vi "PicoScope3000aExampleBlockMSO_MultipleDevices.vi"() -> ()   [LabVIEW 2010]
uses:
  shared/PicoBuffers.ctl
  shared/Buffer and Transfer Settings.ctl
  shared/Acquisition Settings.ctl
  PicoScope3000aLib/PicoScope3000aDigitalChannelSettings.ctl
  PicoScope3000aLib/PicoScope3000aAnalogChannelSettings.ctl
panel:
  out "Overflow":i16[](array[numeric])
  in  "Serial Numbers":string[](array[string])
  out "Device Info":T1(array[cluster])
  out "Properties panel":T2(array[cluster]) {"Sample Frequency" format="%#_4p"; "Sample Rate" format="%#_4p"; "Max Samples Available" format="%#_4p"; "Number of Samples" format="%#_4p"; "Total Capture Time (sec)" format="%#_4p"; "Max Total Capture Time Available (sec)" format="%#_4p"}
  in  "Use Serial Numbers":bool
  in  "Scope Index":i32
  in  "Trigger Settings":T3={"Trigger Enabled"=FALSE, "Trigger Source"=enum."Channel A", "Trigger Threshold (volts)"=0.0, "Trigger Direction"=2, "Trigger Delay (samples)"=0, "Auto Trigger Time (ms)"=1000} {"Trigger Direction" items=["Above", "Below", "Rising", "Falling", "Rising or Falling"]}
  in  "Channel A Settings":T4={"Enabled"=TRUE, "Coupling"=1, "Range"=6, "Analogue Offset"=0.0, "Bandwidth Limit"=0} {"Bandwidth Limit" items=["Full", "20MHz"]; "Range" items=["10 mV", "20 mV", "50 mV", "100 mV", "200 mV", "500 mV", "1 V", "2 V", "5 V", "10 V", "20 V", "50 V ", "100 V"]; "Coupling" items=["AC", "DC"]}
  in  "Port 0 Settings":T5={"Enabled"=FALSE, "Logic Level"=9830} {"Logic Level" items=["1.5V TTL"=9830, "2.5V CMOS"=16383]}
  in  "Apply Settings":bool
  out "USB 3.0 device on non-USB 3.0 Port":bool=TRUE
  out "USB Powered":bool=TRUE
  out "error out":errorcluster
  in  "Buffer and Transfer Settings":T6={"startIndex"=0, "Samples"=100000, "Down Sample Ratio"=1, "Down-Sample Mode"=0} {"Down-Sample Mode" items=["RAW none"=2147483648, "None"=0, "Aggregate"=1, "Decimate"=2, "Average"=4]; "Down Sample Ratio" step=1; "Samples" format="%_6p"}
  in  "Acquisition Settings":T7={"preTriggerSamples"=0, "postTriggerSamples"=100000, "timebase"=10} {"postTriggerSamples" format="%_6p"; "preTriggerSamples" format="%_6p"}
  in  "stop":bool
  out "Scope \"N\"":cluster{i32, sgl, "Data":dbl[]}[](graph)
  in  "error in (no error)":errorcluster
  # "Bit 0 = ChA"
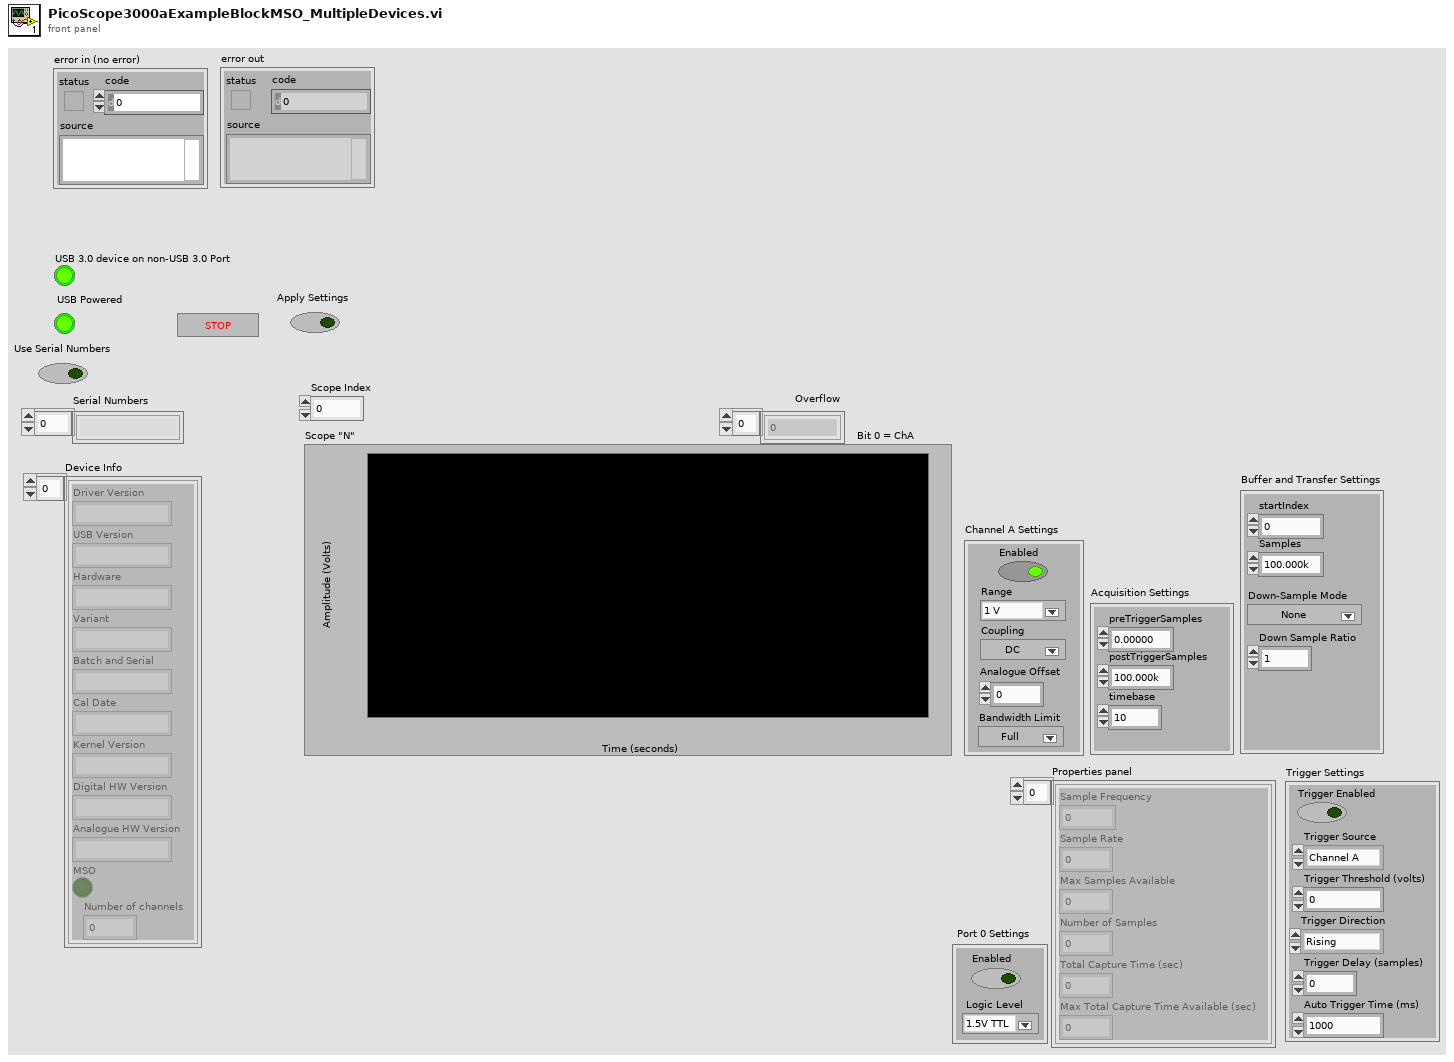
[diagram p1: front panel]
types:
  T1 = cluster{"Driver Version":string, "USB Version":string, "Hardware":string, "Variant":string, "Batch and Serial":string, "Cal Date":string, "Kernel Version":string, "Digital HW Version":string, "Analogue HW Version":string, "MSO":bool, "Number of channels":i16}[]
  T2 = cluster{"Sample Frequency":sgl, "Sample Rate":sgl, "Max Samples Available":i32, "Number of Samples":u32, "Total Capture Time (sec) ":sgl, "Max Total Capture Time Available (sec)":sgl}[]
  T3 = cluster{"Trigger Enabled":bool, "Trigger Source":enum32{"Channel A", "Channel B", "Channel C", "Channel D", "Ext."}, "Trigger Threshold (volts)":dbl, "Trigger Direction":u32, "Trigger Delay (samples)":u32, "Auto Trigger Time (ms)":i16}
  T4 = typedef "PicoScope3000aAnalogChannelSettings.ctl" = cluster{"Enabled":bool, "Coupling":u32, "Range":u32, "Analogue Offset":sgl, "Bandwidth Limit":u32}
  T5 = typedef "PicoScope3000aDigitalChannelSettings.ctl" = cluster{"Enabled":bool, "Logic Level":i16}
  T6 = typedef "Buffer and Transfer Settings.ctl" = cluster{"startIndex":u64, "Samples":u64, "Down Sample Ratio":u64, "Down-Sample Mode":u32}
  T7 = typedef "Acquisition Settings.ctl" = cluster{"preTriggerSamples":u64, "postTriggerSamples":u64, "timebase":u32}
  T8 = typedef "PicoBuffers.ctl" = cluster{"Max Buffer Pointers":u64[][][], "Min Buffer Pointers":u64[][][], "StreamingDataInfo":cluster{"Channel":u32, "Down-Sample Mode":u32, "PICO_DATA_TYPE":enum32{"PICO_INT8_T", "PICO_INT16_T", "PICO_INT32_T", "PICO_UINT32_T", "PICO_INT64_T", ""}, "Samples":i32, "bufferIndex":u64, "startIndex":i32, "overflow":i16}[][]}
  T9 = cluster{"Driver Version":string, "USB Version":string, "Hardware":string, "Variant":string, "Batch and Serial":string, "Cal Date":string, "Kernel Version":string, "Digital HW Version":string, "Analogue HW Version":string, "MSO":bool, "Number of channels":i16}
  T10 = cluster{"Sample Frequency":sgl, "Sample Rate":sgl, "Max Samples Available":i32, "Number of Samples":u32, "Total Capture Time (sec) ":sgl, "Max Total Capture Time Available (sec)":sgl}
  T11 = cluster{"Channel A Buffer":i16[], "Channel B Buffer":i16[], "Channel C Buffer":i16[], "Channel D Buffer":i16[], "Channel E Buffer":i16[], "Channel F Buffer":i16[], "Channel G Buffer":i16[], "Channel H Buffer":i16[], "Port 0 Buffer":i16[], "Port 1 Buffer":i16[]}[]
  T12 = cluster{"Channel A Buffer":i16[], "Channel B Buffer":i16[], "Channel C Buffer":i16[], "Channel D Buffer":i16[], "Channel E Buffer":i16[], "Channel F Buffer":i16[], "Channel G Buffer":i16[], "Channel H Buffer":i16[], "Port 0 Buffer":i16[], "Port 1 Buffer":i16[]}
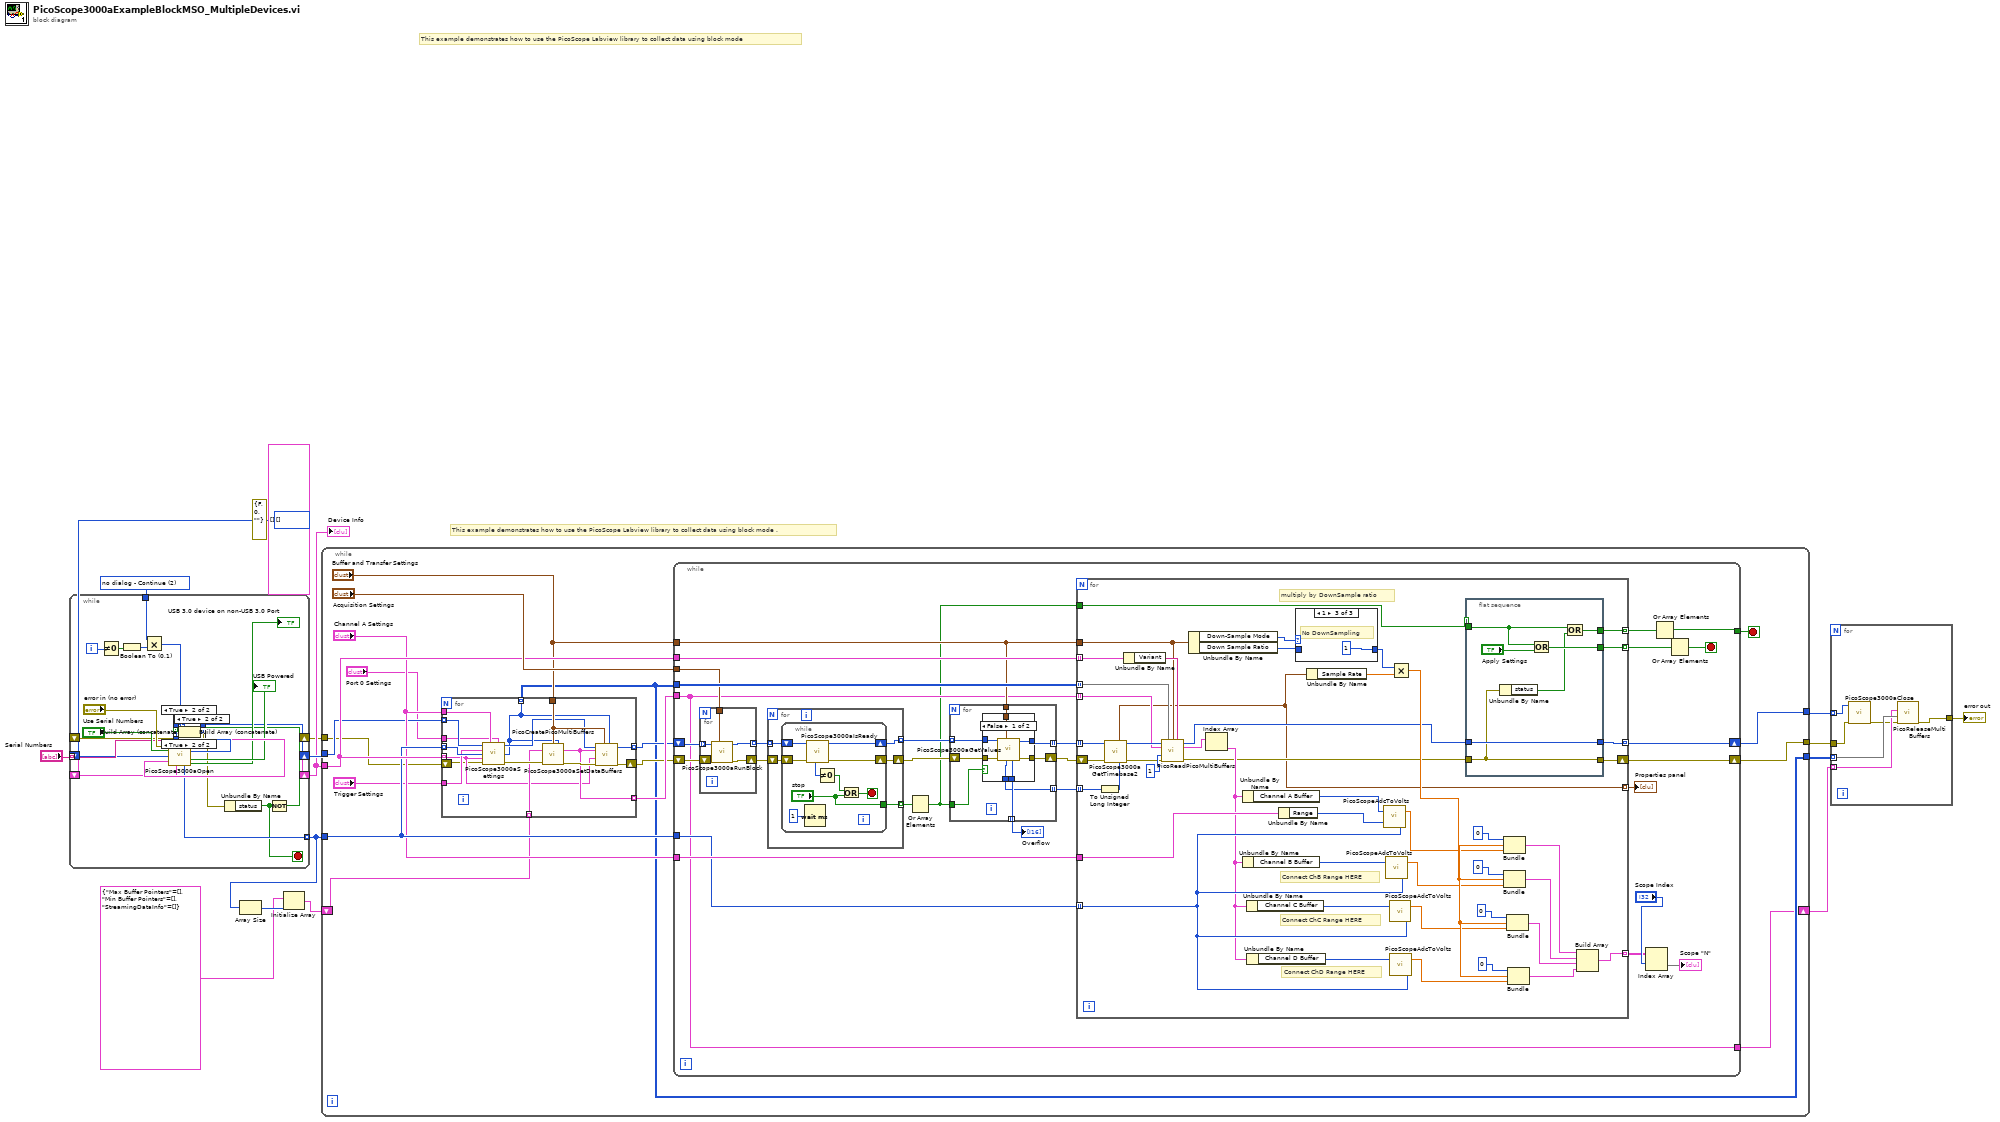
[diagram p0: block diagram]
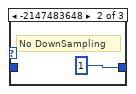
[diagram p6: hidden frame]
diagram:
  w9 = u16 2 items=["Dialog On Error", "no dialog - CloseUnit and Stop", "no dialog - Continue", "no dialog - Stop"] ("Mode")
  # "This example demonstrates how to use the PicoScope Labview library to collect data using block mode ."
  # "This example demonstrates how to use the PicoScope Labview library to collect data using block mode"
  n1 = while {
    tunnel: [w35] -> w6 mode=indexing
    tunnel: w9 -> [w30]
    tunnel: "Serial Numbers" -> [w24] mode=indexing
    shift-right: [w22] -> w17
    shift-left: i16[] [] ("Array") -> [w23]
    shift-right: [w20] -> w15
    shift-left: T1 [] ("Array") -> [w21]
    shift-right: [w18] -> w14
    shift-left: errorcluster {"status"=FALSE, "code"=0, "source"=""} ("error out 2") -> [w19]
    i -> [w31]
    stop <- w27 stop-if-true
    n2 = Not Equal To 0?(x=w31) -> (x != 0?=w33:bool)
    n3 = Boolean To (0,1)(Boolean=w33) -> (0, 1=w32:i16)
    n4 = Multiply(x=w30, y=w32) -> (x*y=w29:u16)
    n5 = call "PicoScope3000aOpen.vi"("error in (no error)"="error in (no error)", "Serial Number"=w24, "Mode"=w29, "Use Serial number"="Use Serial Numbers") -> ("error out"=w28:errorcluster, "handle"=w39:i16, "USB Powered"=→"USB Powered":bool, "Device Info"=w37:T9, "Max ADC value"=w35:i16, "USB 3.0 device on non-USB 3.0 Port"=→"USB 3.0 device on non-USB 3.0 Port":bool)  [unwired: 5 in, 1 out]
    n6 = Unbundle By Name(w28) -> ("status"=w27:bool)
    n7 = Not(x=w27) -> (.not. x?=w26:bool)
    n8 = case shown="True" w26 {
      tunnel: w19 -> [w40 _]
      tunnel: w28 -> [_ w41]
      tunnel: [w40 w41] -> w18
      frame False {
      }
      frame True {
      }
    }
    n9 = case shown="True" w26 {
      tunnel: w21 -> [w42 w44]
      tunnel: w37 -> [_ w43]
      tunnel: [w42 w45] -> w20
      frame False {
      }
      frame True {
        n10 = Build Array (concatenate)(w44, w43) -> (w45:T1)
      }
    }
    n11 = case shown="True" w26 {
      tunnel: w23 -> [w46 w48]
      tunnel: w39 -> [_ w47]
      tunnel: [w46 w49] -> w22
      frame False {
      }
      frame True {
        n12 = Build Array (concatenate)(w48, w47) -> (w49:i16[])
      }
    }
  }
  "Device Info" <- w15
  n13 = Array Size(array=w6) -> (size(s)=w8:i32)
  n14 = Initialize Array(T8 {"Max Buffer Pointers"=[], "Min Buffer Pointers"=[], "StreamingDataInfo"=[]} ("Data Pointers"), w8) -> (w7:T8[])
  n15 = while {
    tunnel: w17 -> [w57]
    tunnel: w6 -> [w59]
    tunnel: [w54] -> w16
    tunnel: w15 -> [w65]
    tunnel: w14 -> [w56]
    tunnel: [w64] -> w13
    tunnel: [w63] -> w12
    shift-right: [w50] -> w10
    shift-left: w7 -> [w51]
    stop <- w52 stop-if-true
    n16 = for {
      tunnel: w65 -> [w69] mode=indexing
      tunnel: "Buffer and Transfer Settings" -> [w80]
      tunnel: "Channel A Settings" -> [w78]
      tunnel: w57 -> [w77] mode=indexing
      tunnel: "Trigger Settings" -> [w76]
      tunnel: [w74] -> w54 mode=indexing
      tunnel: "Port 0 Settings" -> [w72]
      shift-right: [w82] -> w62
      shift-left: w56 -> [w68]
      tunnel: w59 -> [w79] mode=indexing
      tunnel: [w81] -> w61 mode=indexing
      tunnel: [w71] -> w67 mode=indexing
      tunnel: w51 -> [w70] mode=indexing
      n17 = call "PicoScope3000aSettings.vi"("handle in"=w77, "Channel A Settings"=w78, "Port 0 Settings"=w72, "Trigger Settings"=w76, "Max_adc"=w79, "Device Info"=w69, "error in"=w68) -> ("handle out"=w75:i16, "Enabled Array"=w74:i16[], "error out"=w73:errorcluster)  [unwired: 6 in]
      n18 = call "PicoCreatePicoMultiBuffers.vi"("Buffer and Transfer Settings"=w80, "enabled array"=w74, "Data Pointers In"=w70, "error in (no error)"=w73) -> ("Data Pointers"=w71:T8, "error out"=w83:errorcluster)  [unwired: 10 in]
      n19 = call "PicoScope3000aSetDataBuffers.vi"("enabled array"=w74, "Buffer and Transfer Settings"=w80, "error in (no error)"=w83, "Device Info"=w69, "Data Pointers In"=w71, "handle in"=w75) -> ("error out"=w82:errorcluster, "handle out"=w81:i16)  [unwired: 4 in]
    }
    n20 = while {
      tunnel: w67 -> [w88]
      tunnel: "Buffer and Transfer Settings" -> [w99]
      tunnel: w54 -> [w110]
      tunnel: "Channel A Settings" -> [w109]
      tunnel: "Acquisition Settings" -> [w108]
      tunnel: w59 -> [w107]
      tunnel: w65 -> [w106]
      shift-right: [w105] -> w64
      shift-left: w62 -> [w100]
      shift-right: [w104] -> w63
      shift-left: w61 -> [w101]
      tunnel: [w92] -> w52
      tunnel: [w88] -> w50
      stop <- w91 stop-if-true
      n21 = for {
        tunnel: [w203] -> w111 mode=indexing
        tunnel: w108 -> [w202]
        tunnel: w101 -> [w201] mode=indexing
        shift-right: [w204] -> w112
        shift-left: w100 -> [w200]
        n22 = call "PicoScope3000aRunBlock.vi"("Acquisition Settings"=w202, "error in (no error)"=w200, "handle in"=w201) -> ("error out"=w204:errorcluster, "handle out"=w203:i16)  [unwired: 5 in, 2 out]
      }
      n23 = for {
        tunnel: w111 -> [w189] mode=indexing
        tunnel: [w188] -> w103 mode=indexing
        tunnel: [w186] -> w87 mode=indexing
        shift-right: [w187] -> w102
        shift-left: w112 -> [w190]
        n24 = while {
          shift-right: [w198] -> w187
          shift-left: w190 -> [w199]
          shift-right: [w197] -> w188
          shift-left: w189 -> [w196]
          tunnel: ["stop"] -> w186
          stop <- w193 stop-if-true
          n25 = Wait (ms)(milliseconds to wait=u32 1) -> ()  [unwired: 1 out]
          n26 = call "PicoScope3000aIsReady.vi"("error in (no error)"=w199, "handle in"=w196) -> ("error out"=w198:errorcluster, "handle out"=w197:i16, "ready"=w195:i16)  [unwired: 7 in]
          n27 = Not Equal To 0?(x=w195) -> (x != 0?=w194:bool)
          n28 = Or(x=w194, y="stop") -> (x .or. y?=w193:bool)
        }
      }
      n29 = Or Array Elements(Boolean array=w87) -> (logical OR=w86:bool)
      n30 = for {
        tunnel: w103 -> [w176] mode=indexing
        tunnel: w99 -> [w174]
        tunnel: w86 -> [w173]
        tunnel: [w172] -> w84 mode=indexing
        tunnel: [w170] -> w97 mode=indexing
        tunnel: [w169] -> w96 mode=indexing
        shift-right: [w171] -> w98
        shift-left: w102 -> [w175]
        n31 = case shown="False" w173 {
          tunnel: w175 -> [w183 w184]
          tunnel: w176 -> [w182 w185]
          tunnel: [w181 w185] -> w170
          tunnel: [w180 w184] -> w171
          tunnel: w174 -> [w179 _]
          tunnel: [w178 _] -> w172
          tunnel: [w177 _] -> w169
          frame False {
            n32 = call "PicoScope3000aGetValues.vi"("Buffer and Transfer Settings"=w179, "error in (no error)"=w183, "handle in"=w182) -> ("error out"=w180:errorcluster, "handle out"=w181:i16, "overflow"=w178:i16, "noOfSamples"=w177:u64)  [unwired: 5 in]
          }
          frame True {
          }
        }
      }
      "Overflow" <- w84
      n33 = for {
        tunnel: w88 -> [w115] mode=indexing
        tunnel: w110 -> [w153] mode=indexing
        tunnel: w109 -> [w152]
        tunnel: w107 -> [w151] mode=indexing
        tunnel: w106 -> [w148] mode=indexing
        tunnel: [w139] -> w89 mode=indexing
        tunnel: [w125] -> w90 mode=indexing
        tunnel: [w124] -> w104 mode=indexing
        tunnel: w99 -> [w123]
        tunnel: w97 -> [w121] mode=indexing
        tunnel: w96 -> [w118] mode=indexing
        shift-right: [w127] -> w105
        shift-left: w98 -> [w122]
        tunnel: w86 -> [w114]
        tunnel: [w116] -> w93 mode=indexing
        tunnel: [w113] -> w85 mode=indexing
        # "Connect ChB Range HERE"
        # "Connect ChD Range HERE"
        # "Connect ChC Range HERE"
        # "multiply by DownSample ratio"
        n34 = To Unsigned Long Integer(number=w118) -> (unsigned 32bit integer=w117:u32)
        n35 = call "PicoScope3000aGetTimebase2.vi"("Number of Samples"=w117, "error in (no error)"=w122, "handle in"=w121) -> ("error out"=w120:errorcluster, "handle out"=w119:i16, "Properties Panel"=w113:T10)  [unwired: 6 in]
        n36 = Unbundle By Name(w148) -> ("Variant"=w149:string)
        n37 = call "PicoReadPicoMultiBuffers.vi"("enabled array"=w153, "Buffer and Transfer Settings"=w123, "Variant"=w149, "Data Pointers"=w115, "No of Buffers"=1, "error in (no error)"=w120) -> ("MultiBuffers (Max or non-aggregated)"=w158:T11, "error out"=w126:errorcluster)  [unwired: 7 in, 1 out]
        n38 = Unbundle By Name(w123) -> ("Down-Sample Mode"=w156:u32, "Down Sample Ratio"=w157:u64)
        n39 = Index Array(array=w158) -> (element=w128:T12)  [unwired: 1 in]
        n40 = Unbundle By Name(w128) -> ("Channel A Buffer"=w137:i16[])
        n41 = Unbundle By Name(w128) -> ("Channel B Buffer"=w143:i16[])
        n42 = Unbundle By Name(w128) -> ("Channel C Buffer"=w135:i16[])
        n43 = Unbundle By Name(w128) -> ("Channel D Buffer"=w131:i16[])
        n44 = Unbundle By Name(w152) -> ("Range"=w145:u32)
        n45 = case shown="1" w156 {
          tunnel: [w166 u64 1 ("Down Sample Ratio") u64 1 ("Down Sample Ratio")] -> w154
          tunnel: w157 -> [w166 _ _]
          frame Default {
          }
          frame -2147483648 {
            # "No DownSampling"
          }
          frame 1 {
            # "No DownSampling"
          }
        }
        n46 = Unbundle By Name(w113) -> ("Sample Rate"=w150:sgl)
        n47 = call "PicoScopeAdcToVolts.vi"("Max_adc"=w151, "Range Index"=w145, "Data"=w137) -> ("Data"=w138:dbl[])
        n48 = call "PicoScopeAdcToVolts.vi"("Max_adc"=w151, "Data"=w143) -> ("Data"=w142:dbl[])  [unwired: 1 in]
        n49 = call "PicoScopeAdcToVolts.vi"("Max_adc"=w151, "Data"=w135) -> ("Data"=w134:dbl[])  [unwired: 1 in]
        n50 = call "PicoScopeAdcToVolts.vi"("Max_adc"=w151, "Data"=w131) -> ("Data"=w130:dbl[])  [unwired: 1 in]
        n51 = Multiply(x=w154, y=w150) -> (x*y=w155:sgl)
        n52 = flat-sequence {
          tunnel: [w165] -> w125
          tunnel: w114 -> [w159]
          tunnel: [w162] -> w116
          tunnel: w119 -> [w161]
          tunnel: [w161] -> w124
          tunnel: w126 -> [w160]
          tunnel: [w160] -> w127
          frame #0 {
            n53 = Unbundle By Name(w160) -> ("status"=w163:bool)
            n54 = Or(x=w159, y="Apply Settings") -> (x .or. y?=w165:bool)
            n55 = Or(x=w159, y=w163) -> (x .or. y?=w162:bool)
          }
        }
        n56 = Bundle(0, w155, "Data"=w138) -> (w141:cluster{i32, sgl, "Data":dbl[]})  [unwired: 1 in]
        n57 = Bundle(0, w155, "Data"=w142) -> (w140:cluster{i32, sgl, "Data":dbl[]})  [unwired: 1 in]
        n58 = Bundle(0, w155, "Data"=w134) -> (w133:cluster{i32, sgl, "Data":dbl[]})  [unwired: 1 in]
        n59 = Bundle(0, w155, "Data"=w130) -> (w129:cluster{i32, sgl, "Data":dbl[]})  [unwired: 1 in]
        n60 = Build Array(w141, w140, w133, w129) -> (w139:cluster{i32, sgl, "Data":dbl[]}[])
      }
      "Properties panel" <- w85
      n61 = Index Array(array=w89, index (row)="Scope Index") -> (element=→"Scope \"N\"":cluster{i32, sgl, "Data":dbl[]}[])  [unwired: 1 in]
      n62 = Or Array Elements(Boolean array=w93) -> (logical OR=w92:bool)
      n63 = Or Array Elements(Boolean array=w90) -> (logical OR=w91:bool)
    }
  }
  n64 = for {
    tunnel: w16 -> [w210] mode=indexing
    tunnel: w13 -> [w206]
    tunnel: w12 -> [w209] mode=indexing
    tunnel: [w208] -> w11
    tunnel: w10 -> [w207] mode=indexing
    n65 = call "PicoScope3000aClose.vi"("error in (no error)"=w206, "handle in"=w209) -> ("error out"=w205:errorcluster)  [unwired: 8 in, 1 out]
    n66 = call "PicoReleaseMultiBuffers.vi"("error in (no error)"=w205, "Enabled array"=w210, "Data Pointers"=w207) -> ("error out"=w208:errorcluster)  [unwired: 7 in, 1 out]
  }
  "error out" <- w11
